vi "Set File Attributes.vi"(6 "timeout (ms)":i32=30000, 8 "error in":errorcluster, 9 "file attributes":refnum<class "File Attributes.lvclass">, 10 "remote path":string, 11 "session in":refnum<class "Session.lvclass">) -> (0 "error out":errorcluster, 3 "session out":refnum<class "Session.lvclass">)   [LabVIEW 2020, in "NI_SFTP.lvlib"]
doc: "Update mutable information about a remote file or directory, including modification time and file size."
uses:
  <vilib>/net/SFTP/NI_SFTP.lvlib
  <vilib>/net/SFTP/Session/Session.lvclass
  <vilib>/net/SFTP/File Attributes/File Attributes.lvclass
  <vilib>/net/SFTP/File Attributes/File Attributes.lvclass/File Attributes.ctl
  <vilib>/net/SFTP/API/Support/Command/SSH_FXP_SETSTAT/Input.ctl
  <vilib>/net/SFTP/API/Support/File Attributes.ctl
  <vilib>/Utility/Deadline/NI_Deadline.lvlib
  <vilib>/net/SFTP/API/Support/Command/SSH_FXP_SETSTAT/SSH_FXP_SETSTAT.lvclass
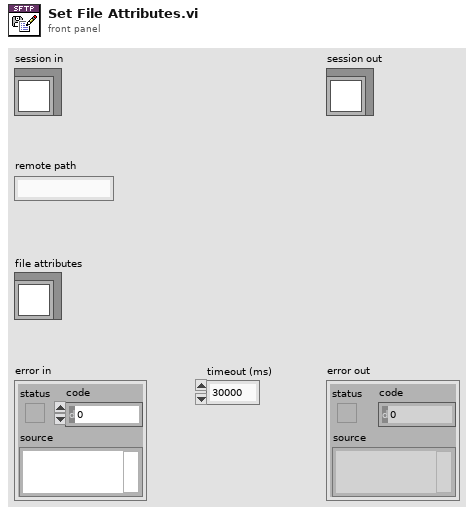
[diagram p1: front panel]
types:
  T1 = typedef "NI_SFTP.lvlib/SSH_FXP_SETSTAT.lvclass/Input.ctl" = cluster{"path":string, "file attributes":T2}
  T2 = typedef "NI_SFTP.lvlib/File Attributes.ctl" = cluster{"SSH_FILEXFER_ATTR_SIZE":bool, "size":u64, "SSH_FILEXFER_ATTR_UIDGID":bool, "uid":u32, "gid":u32, "SSH_FILEXFER_ATTR_PERMISSIONS":bool, "permissions":u32, "SSH_FILEXFER_ATTR_ACMODTIME":bool, "atime":u32, "mtime":u32, "extended":map{string, string}}
  T3 = typedef "NI_Deadline.lvlib/Deadline.ctl" = cluster{"mode":T4, "deadline (ms)":u32}
  T4 = typedef "NI_Deadline.lvlib/Mode.ctl" = enum16{"Relative", "Use deadline", "Wait forever", "Nonblocking", "N/A"}
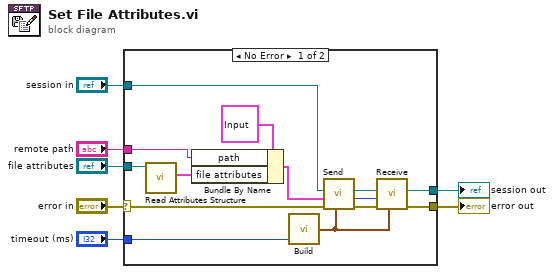
[diagram p0: block diagram]
diagram:
  n1 = case shown="No Error" "error in" {
    selector: "error in" -> [w21 w23]
    tunnel: [w18 w23] -> w4
    tunnel: [w13 w22] -> w5
    tunnel: "session in" -> [w8 w22]
    tunnel: "remote path" -> [w11 _]
    tunnel: "timeout (ms)" -> [w20 _]
    tunnel: "file attributes" -> [w16 _]
    frame No Error {
      n2 = call <vilib>:"Read Attributes Structure.vi"("file attributes in"=w16) -> ("file attributes"=w10:T2)  [unwired: 9 in, 1 out]
      n3 = Bundle By Name(cluster=T1 {"path"="", "file attributes"={"SSH_FILEXFER_ATTR_SIZE"=FALSE, "size"=0, "SSH_FILEXFER_ATTR_UIDGID"=FALSE, "uid"=0, "gid"=0, "SSH_FILEXFER_ATTR_PERMISSIONS"=FALSE, "permissions"=0, "SSH_FILEXFER_ATTR_ACMODTIME"=FALSE, "atime"=0, "mtime"=0, "extended"={}}} ("input"), "path"=w11, "file attributes"=w10) -> (w9:T1)
      n4 = call <vilib>:"Build.vi"("timeout (ms)"=w20) -> ("Deadline out"=w17:T3)  [unwired: 2 in]
      n5 = call <vilib>:"Send.vi"("deadline"=w17, "error in (no error)"=w21, "input"=w9, "session in"=w8) -> ("error out"=w19:errorcluster, "request id"=w15:u32, "session out"=w14:refnum<class "Session.lvclass">)  [unwired: 4 in, 1 out]
      n6 = call <vilib>:"Receive.vi"("deadline"=w17, "error in (no error)"=w19, "request id"=w15, "session in"=w14) -> ("error out"=w18:errorcluster, "session out"=w13:refnum<class "Session.lvclass">)  [unwired: 4 in, 2 out]
    }
    frame Error {
    }
  }
  "error out" <- w4
  "session out" <- w5
